vi "TubingCompensation.vi"(7 "NyquistLimitedCoefficients":dbl[](array[numeric]), 10 "mutedData":dbl[](array[numeric]), 11 "SamplingFreq":dbl) -> (2 "boostedData":dbl[](array[numeric]))   [LabVIEW 2011]
uses:
  <vilib>/Analysis/NI_AALBase.lvlib
panel:
  out "SDincrease(%)":dbl
  out "meanDifference":dbl format="%.2e"
  out "Waveform Graph":dbl[][](graph)
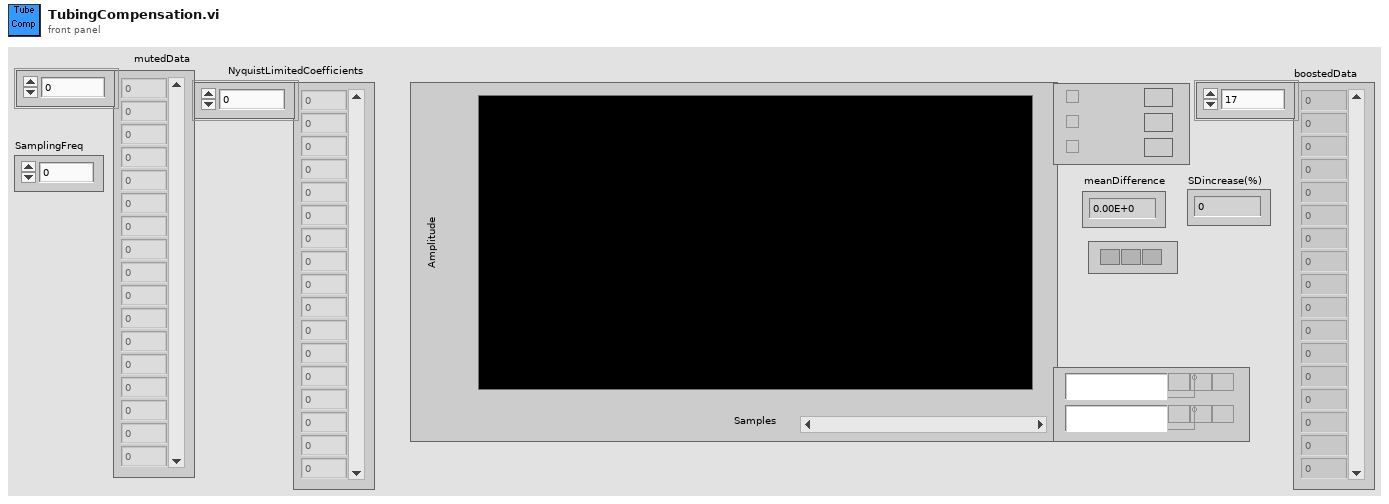
[diagram p1: front panel]
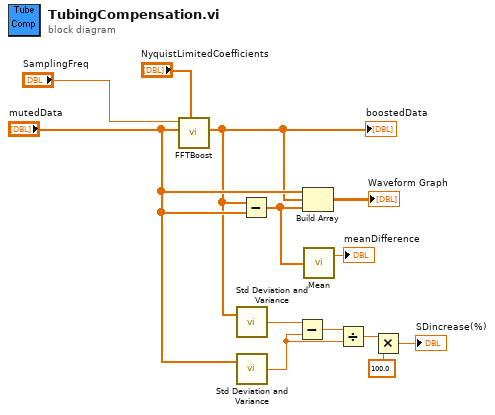
[diagram p0: block diagram]
diagram:
  n1 = call "FFTBoost.vi"("CompensationCoefficients"="NyquistLimitedCoefficients", "mutedData"="mutedData", "SamplingFreq (for graph)"="SamplingFreq") -> ("boostedData"=w7:dbl[])  [unwired: 1 in, 7 out]
  "boostedData" <- w7
  n2 = call <vilib>:"Std Deviation and Variance.vi"("X"=w7) -> ("standard deviation"=w6:dbl)  [unwired: 1 in, 2 out]
  n3 = call <vilib>:"Std Deviation and Variance.vi"("X"="mutedData") -> ("standard deviation"=w4:dbl)  [unwired: 1 in, 2 out]
  n4 = Subtract(x=w7, y="mutedData") -> (x-y=w10:dbl[])
  n5 = Subtract(x=w6, y=w4) -> (x-y=w5:dbl)
  n6 = Build Array("mutedData", w7, w10) -> (→"Waveform Graph":dbl[][])
  n7 = call <vilib>:"Mean.vi"("X"=w10) -> ("mean"=→"meanDifference":dbl)  [unwired: 1 out]
  n8 = Divide(x=w5, y=w4) -> (x/y=w3:dbl)
  n9 = Multiply(x=w3, y=100.0) -> (x*y=→"SDincrease(%)":dbl)
